vi "Pre Launch Init.vi"(11 "Nested in":refnum<class "UI_Up_Down.lvclass">) -> (0 "error out":errorcluster, 3 "Nested out":refnum<class "UI_Up_Down.lvclass">)   [LabVIEW 2021, in "UI_Up_Down.lvclass"]
doc: "(<B>Filename</B>: Actor Framework.lvlib:Actor.lvclass:Pre Launch Init.vi)\n\nDefines behavior that occurs after the Launch Nested Actor method is invoked but before the actor's Actor Core method begins running.\n\nBy default, this method does nothing. A descendant class may override it to define behavior."
uses:
  UI_Up_Down.lvclass
  UI_Up_Down.lvclass/UI_Up_Down.ctl
  <userlib>/John_Lib/AbstractActorTemplate/AbstractActorTemplate/UIActorTop.lvclass
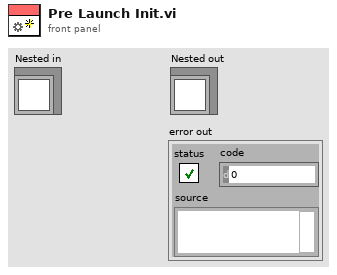
[diagram p1: front panel]
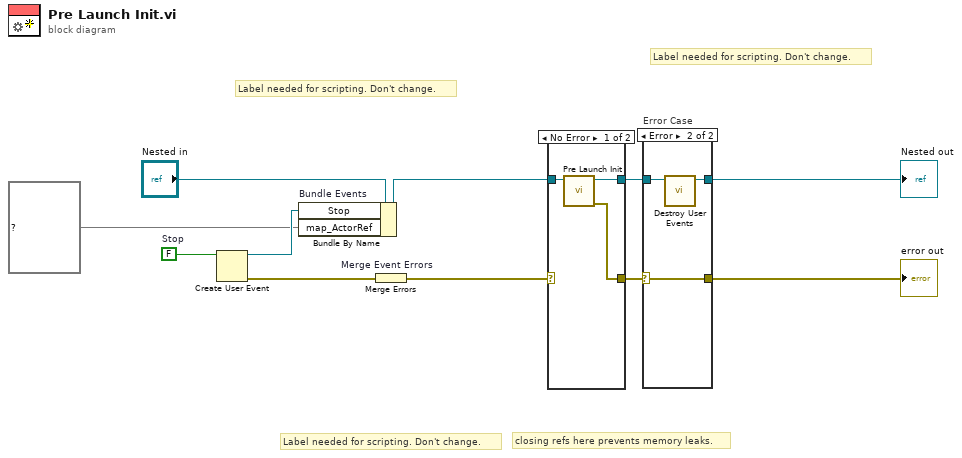
[diagram p0: block diagram]
diagram:
  w10 = FALSE  # Stop
  # "Label needed for scripting. Don't change."
  # "Label needed for scripting. Don't change."
  # "Label needed for scripting. Don't change."
  # "closing refs here prevents memory leaks."
  n1 = Create User Event(user event datatype=w10) -> (user event=w7:refnum<user-event>, error out=w9:errorcluster)  [unwired: 1 in]
  n2 = Bundle By Name "Bundle Events"(cluster="Nested in", "Stop"=w7, "map_ActorRef"=map{string, refnum<vi>} {}) -> (w4:refnum<class "UI_Up_Down.lvclass">)
  n3 = Merge Errors "Merge Event Errors"(w9) -> (w3:errorcluster)
  n4 = case shown="No Error" w3 {
    selector: w3 -> [_ w16]
    tunnel: [w14 w15] -> w5
    tunnel: w4 -> [w13 w15]
    tunnel: [w12 w16] -> w2
    frame No Error {
      n5 = call-parent "Pre Launch Init.vi"("Actor in"=w13) -> ("error out"=w12:errorcluster, "Actor out"=w14:refnum<class "UI_Up_Down.lvclass">)  [unwired: 9 in]
    }
    frame Error {
    }
  }
  n6 = case "Error Case" shown="Error" w2 {
    selector: w2 -> [w17 w21]
    tunnel: w5 -> [w18 w20]
    tunnel: [w18 w19] -> w8
    tunnel: [w17 w21] -> w6
    frame No Error {
    }
    frame Error {
      n7 = call "Destroy User Events.vi"("UI Template in"=w20) -> ("UI Template out"=w19:refnum<class "UI_Up_Down.lvclass">)  [unwired: 10 in]
    }
  }
  "error out" <- w6
  "Nested out" <- w8
